vi "Constructor.vi"(6 "Message Queue":refnum<class "Delacor_lib_QMH_Message Queue.lvclass">, 8 "error in (no error)":errorcluster, 9 "Module ID":i32=-1, 10 "Connection ID":refnum<k5>, 11 "GenNet Protocol in":refnum<class "GenNet Protocol.lvclass">) -> (0 "error out":errorcluster, 3 "GenNet Protocol out":refnum<class "GenNet Protocol.lvclass">)   [LabVIEW 2022 SP3, in "hse-gennet.lvlib" / "GenNet Protocol.lvclass"]
doc: "____\nHAMPEL SOFTWARE ENGINEERING v3.8.0 (2023-12-18 14:41)"
uses:
  GenNet Protocol.lvclass
  <vilib>/Delacor/Delacor QMH/Libraries/Message Queue_class/Delacor_lib_QMH_Message Queue.lvclass
  GenNet Protocol.lvclass/GenNet Protocol.ctl
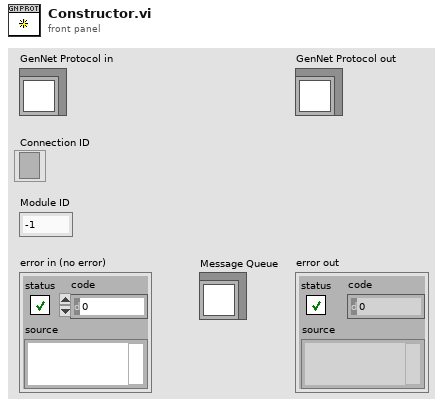
[diagram p1: front panel]
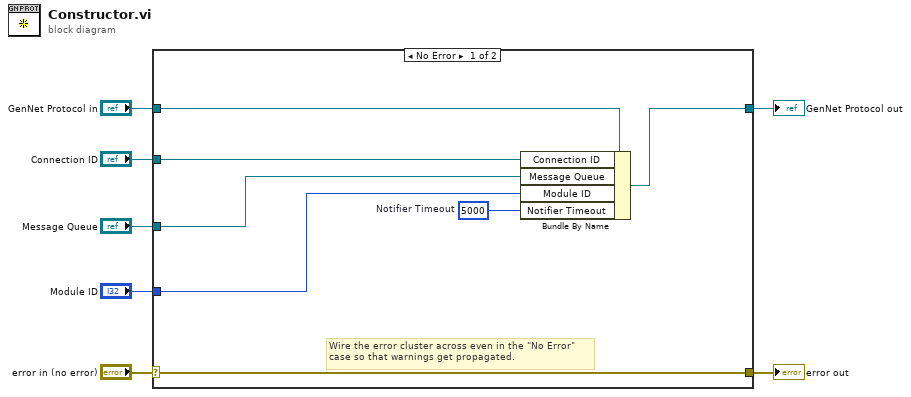
[diagram p0: block diagram]
diagram:
  n1 = case shown="No Error" "error in (no error)" {
    selector: "error in (no error)" -> [w13 w16]
    tunnel: [w13 w16] -> w6
    tunnel: [w12 w15] -> w4
    tunnel: "GenNet Protocol in" -> [w14 w15]
    tunnel: "Connection ID" -> [w11 _]
    tunnel: "Message Queue" -> [w10 _]
    tunnel: "Module ID" -> [w9 _]
    frame No Error {
      w8 = 5000  # Notifier Timeout
      # "Wire the error cluster across even in the \"No Error\"\ncase so that warnings get propagated."
      n2 = Bundle By Name(cluster=w14, "Connection ID"=w11, "Message Queue"=w10, "Module ID"=w9, "Notifier Timeout"=w8) -> (w12:refnum<class "GenNet Protocol.lvclass">)
    }
    frame Error {
    }
  }
  "error out" <- w6
  "GenNet Protocol out" <- w4
